vi "Destroy.vi"(8 "Error In":errorcluster, 11 "Parser":refnum<class "Parser.lvclass">) -> (0 "Error Out":errorcluster)   [LabVIEW 2018, in "Toolkit.lvlib" / "Parser.lvclass"]
uses:
  Parser.lvclass
  Parser.lvclass/Parser.ctl
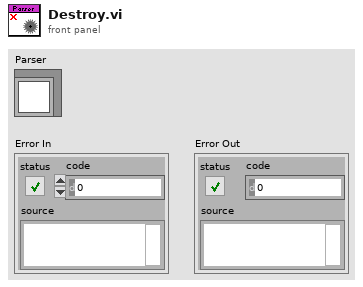
[diagram p1: front panel]
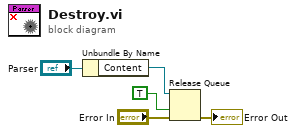
[diagram p0: block diagram]
diagram:
  n1 = Unbundle By Name("Parser") -> ("Content"=w4:refnum<queue>)
  n2 = Release Queue(queue=w4, force destroy? (F)=TRUE, error in (no error)="Error In") -> (error out=→"Error Out":errorcluster)  [unwired: 2 out]
